vi "Write Sequencer State.vi"(8 "error in (no error)":errorcluster, 10 "Sequencer state":T1, 11 "Simple Sequencer in":refnum<class "Simple Sequencer.lvclass">) -> (0 "error out":errorcluster, 3 "Simple Sequencer out":refnum<class "Simple Sequencer.lvclass">)   [LabVIEW 2018, in "Simple Sequencer.lvclass"]
uses:
  Simple Sequencer.lvclass
  NHMFL_Core/Libraries/Instruments/Sequence/Sequencer State Machine/Sequencer State.ctl
  Simple Sequencer.lvclass/Simple Sequencer.ctl
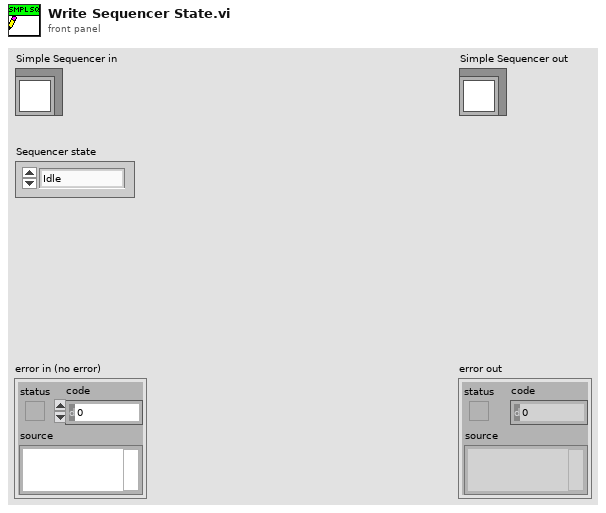
[diagram p1: front panel]
types:
  T1 = typedef "Sequencer State.ctl" = enum16{"Idle", "Starting", "Waiting for primary", "Waiting for secondary"}
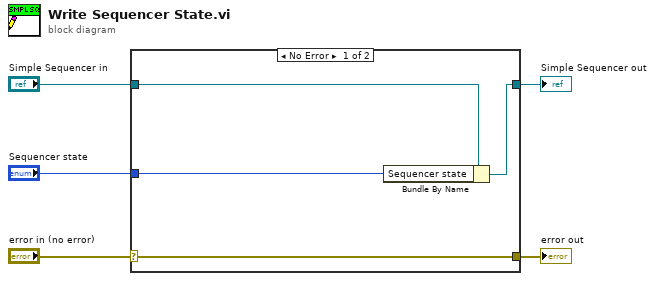
[diagram p0: block diagram]
diagram:
  n1 = case shown="No Error" "error in (no error)" {
    selector: "error in (no error)" -> [w9 w10]
    tunnel: [w9 w10] -> w4
    tunnel: [w7 w11] -> w2
    tunnel: "Simple Sequencer in" -> [w8 w11]
    tunnel: "Sequencer state" -> [w6 _]
    frame No Error {
      n2 = Bundle By Name(cluster=w8, "Sequencer state"=w6) -> (w7:refnum<class "Simple Sequencer.lvclass">)
    }
    frame Error {
    }
  }
  "error out" <- w4
  "Simple Sequencer out" <- w2
